vi "daq test.vi"() -> ()   [LabVIEW 2019]
uses:
  <userlib>/DAQNavi Polymorphic VI/create/DAQNavi Create Channel(AO-Voltage).vi
  <userlib>/DAQNavi Polymorphic VI/create/DAQNavi Create Channel(DO-Digital Output).vi
  <userlib>/DAQNavi Polymorphic VI/create/DAQNavi Create Channel(DI-Digital Input).vi
  <userlib>/DAQNavi Polymorphic VI/write/DAQNavi Write (Analog DBL 1Chan 1Samp).vi
  <userlib>/DAQNavi Polymorphic VI/write/DAQNavi Write (Digtial 1D U8 NChan 1Samp).vi
  <userlib>/DAQNavi Polymorphic VI/read/DAQNavi Read (Digital 1D U8 NChan 1Samp).vi
panel:
  in  "y":dbl
  out "x*y":dbl
  in  "data 2":u8[](array[numeric])
  in  "factor":dbl format="%#_13g"
  in  "bias":dbl
  in  "Numeric":dbl format="%#_13g"
  out "task out digital":i32
  out "task out analog":i32
  out "task out":i32
  out "error out 2":errorcluster
  out "data":u8[](array[numeric])
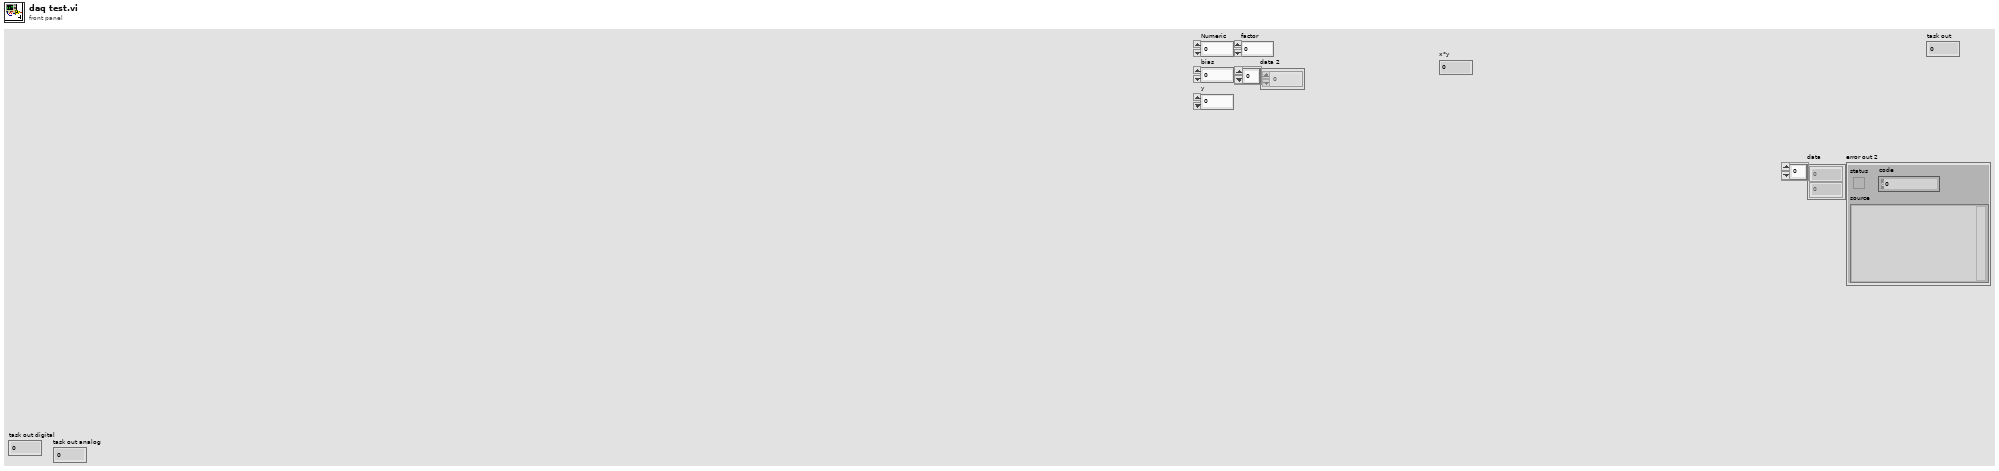
[diagram p1: front panel]
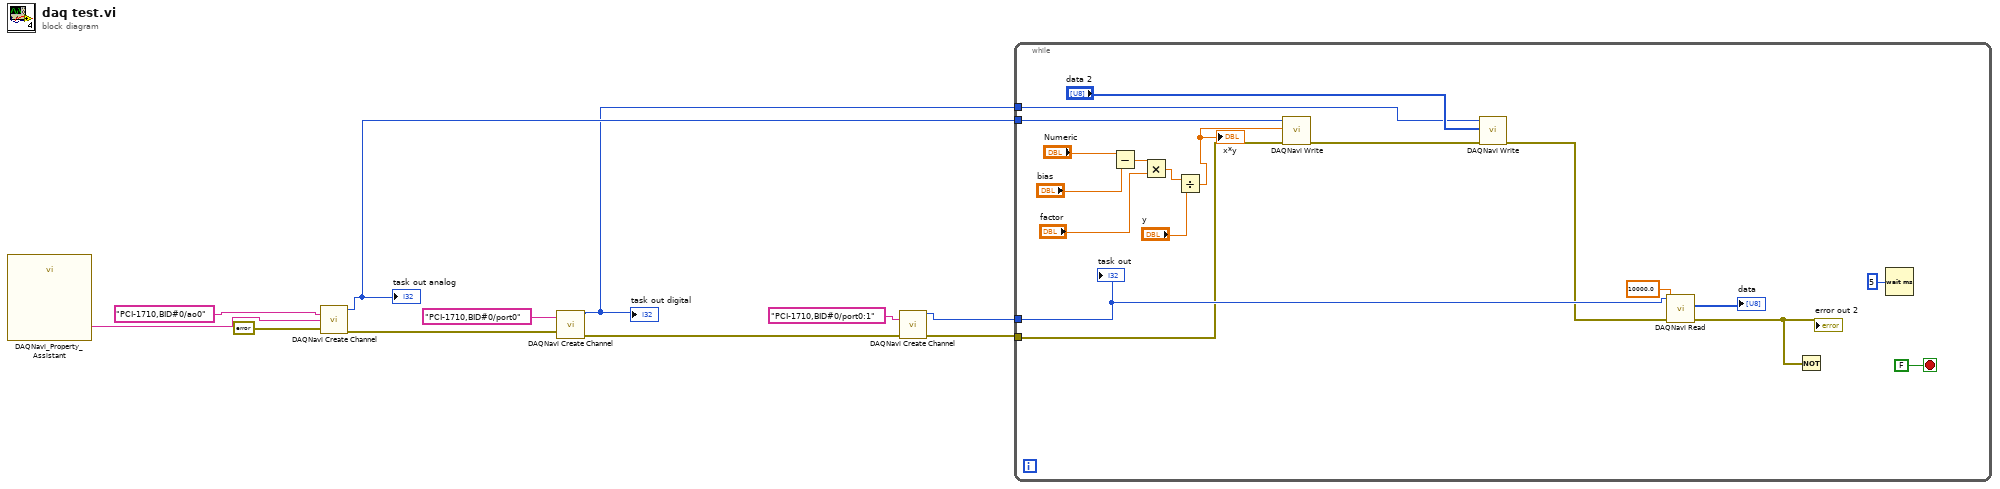
[diagram p0: block diagram]
diagram:
  n1 = call "DAQNavi_Property_Assistant"() -> ("property value"=w8:string)  [unwired: 1 in]
  n2 = call-poly <userlib>:"DAQNavi Create Channel.vi"("physical channels"="PCI-1710,BID#0/ao0", "value range"=w8, "error in (no error)"=errorcluster {"status"=FALSE, "code"=0, "source"=""}) -> ("task out"=w2:i32, "error out"=w9:errorcluster)  [unwired: 11 in]
  "task out analog" <- w2
  n3 = call-poly <userlib>:"DAQNavi Create Channel.vi"("physical channels"="PCI-1710,BID#0/port0", "error in (no error)"=w9) -> ("task out"=w1:i32, "error out"=w11:errorcluster)  [unwired: 12 in]
  "task out digital" <- w1
  n4 = call-poly <userlib>:"DAQNavi Create Channel.vi"("physical channels"="PCI-1710,BID#0/port0:1", "error in (no error)"=w11) -> ("task out"=w3:i32, "error out"=w4:errorcluster)  [unwired: 12 in]
  n5 = while {
    tunnel: w3 -> [w27]
    tunnel: w4 -> [w18]
    tunnel: w2 -> [w25]
    tunnel: w1 -> [w19]
    stop <- FALSE stop-if-true
    n6 = Subtract(x="Numeric", y="bias") -> (x-y=w22:dbl)
    n7 = Multiply(x=w22, y="factor") -> (x*y=w14:dbl)
    n8 = Divide(x=w14, y="y") -> (x/y=w12:dbl)
    "x*y" <- w12
    n9 = call-poly <userlib>:"DAQNavi Write.vi"("error in (no error)"=w18, "data"=w12, "task in"=w25) -> ("error out"=w17:errorcluster)  [unwired: 6 in, 2 out]
    n10 = call-poly <userlib>:"DAQNavi Write.vi"("error in (no error)"=w17, "data"="data 2", "task in"=w19) -> ("error out"=w16:errorcluster)  [unwired: 6 in, 2 out]
    n11 = call-poly <userlib>:"DAQNavi Read.vi"("error in (no error)"=w16, "timeout"=10000.0, "task in"=w27) -> ("error out"=w26:errorcluster, "data"=→"data":u8[])  [unwired: 6 in, 1 out]
    "error out 2" <- w26
    n12 = Not(x=w26) -> ()  [unwired: 1 out]
    n13 = Wait (ms)(milliseconds to wait=u32 5) -> ()  [unwired: 1 out]
    "task out" <- w27
  }
